vi "water level controller.vi"() -> ()   [LabVIEW 2016]
uses:
  <vilib>/LabVIEW Hacker/LINX/Private/Type Defs/Interface.ctl
  <vilib>/MakerHub/LINX/LMH-LINX.lvlib
  <vilib>/MakerHub/LINX/Public/Sensors/Distance/Ultrasonic/Ultrasonic.lvlib
  <vilib>/LabVIEW Hacker/LINX/Private/Type Defs/User Platform.ctl
  <vilib>/MakerHub/LINX/Public/Utilities/Open Serial.vi
panel:
  in  "Lower Tank level":dbl
  in  "Upper Tank Level":dbl
  out "Centimeters":dbl format="%_1f"
  in  "stop":bool
  out "Tank":dbl(slide) scale=0.0..35.0
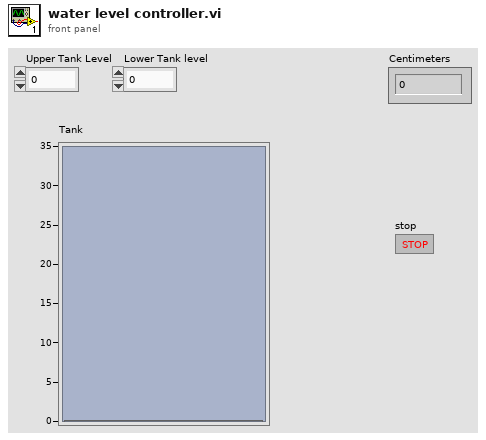
[diagram p1: front panel]
types:
  T1 = typedef "LVH-LINX.lvlib/Interface.ctl" = enum16{"Serial", "TCP"}
  T2 = typedef "LVH-LINX.lvlib/User Platform.ctl" = enum16{"Default", "LINX", "myRIO"}
  T3 = typedef "LMH-LINX.lvlib/LINX Ref.ctl" = cluster{"IO":T4, "Interface":T5, "LINX Device Config":T6}
  T4 = typedef "LMH-LINX.lvlib/Platform.ctl" = enum16{"Remote", "Local"}
  T5 = typedef "LMH-LINX.lvlib/Interface.ctl" = enum16{"Serial", "TCP"}
  T6 = typedef "LMH-LINX.lvlib/Device.lvlib/LINX Device Config.ctl" = cluster{"Interface":T5, "COM Port":refnum<visa-resource-name>, "TCP Configuration":T7, "Device Family":u8, "Device ID":u8, "Device Name":string, "TCP Ref":refnum<k5>, "Channels":T8}
  T7 = typedef "LMH-LINX.lvlib/Device.lvlib/TCP Config.ctl" = cluster{"IP Address":string, "Port":u16}
  T8 = typedef "LMH-LINX.lvlib/Channels.ctl" = cluster{"DI":u8[], "DO":u8[], "AI":u8[], "AO":u8[], "PWM":u8[], "QE":u8[], "UART":u8[], "I2C 2":u8[], "SPI":u8[], "CAN":u8[], "Servo":u8[], "AI Ref (V)":dbl, "AI Resolution (Bits)":u8, "AO Ref (V)":dbl, "AO Resolution (Bits)":u8}
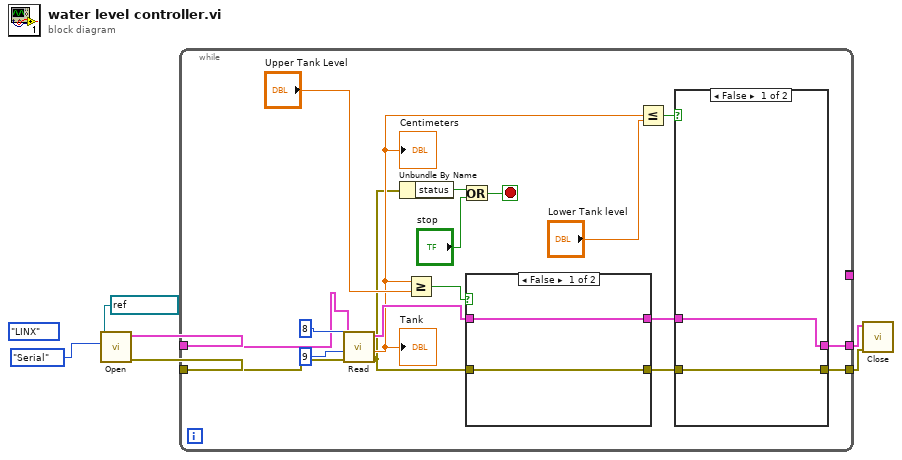
[diagram p0: block diagram]
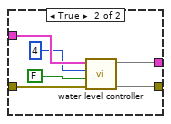
[diagram p2: hidden frame]
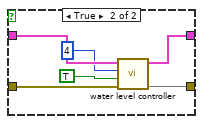
[diagram p3: hidden frame]
diagram:
  (unwired) User_Platform."LINX" ("Platform")
  n1 = call-poly <vilib>:"Open.vi"("Baud Rate Override"=Interface."Serial" ("Interface"), "Serial Port"=refnum<visa-resource-name> "COM23") -> ("Error Out"=w5:errorcluster, "LINX Resource"=w6:T3)  [unwired: 7 in, 1 out]
  n2 = while {
    tunnel: w6 -> [w9]
    tunnel: w5 -> [w8]
    tunnel: [w14] -> w3
    tunnel: [w13] -> w2
    tunnel: [w7] -> _
    tunnel: _ -> [w7]
    stop <- w23 stop-if-true
    n3 = call <vilib>:"Read.vi"("Error In"=w8, "DO Channel"=u8 9 ("Echo Pin (DI)"), "DI Channel"=u8 8 ("Trig"), "LINX Resource"=w9) -> ("Error Out"=w11:errorcluster, "Centimeters"=w12:dbl, "LINX Resource"=w20:T3)  [unwired: 4 in, 1 out]
    "Tank" <- w12
    "Centimeters" <- w12
    n4 = Unbundle By Name(w11) -> ("status"=w25:bool)
    n5 = Greater Or Equal?(x=w12, y="Upper Tank Level") -> (x >= y?=w19:bool)
    n6 = Or(x=w25, y="stop") -> (x .or. y?=w23:bool)
    n7 = case shown="False" w19 {
      tunnel: w20 -> [w35 w41]
      tunnel: w11 -> [w34 w40]
      tunnel: [w35 w37] -> w10
      tunnel: [w34 w36] -> w15
      frame False {
      }
      frame True {
        n8 = call "water level controller.vi"(3:w37, 8:w40, 9:TRUE ("Output Value"), 10:u8 4 ("DO Channel"), 11:w41) -> (0:w36)  [unwired: 6 in]
      }
    }
    n9 = Less Or Equal?(x=w12, y="Lower Tank level") -> (x <= y?=w17:bool)
    n10 = case shown="False" w17 {
      tunnel: w10 -> [w27 w33]
      tunnel: w15 -> [w26 w32]
      tunnel: [w27 w29] -> w14
      tunnel: [w26 w28] -> w13
      frame False {
      }
      frame True {
        n11 = call "water level controller.vi"(8:w32, 9:FALSE ("Output Value"), 10:u8 4 ("DO Channel"), 11:w33) -> (0:w28, 3:w29)  [unwired: 6 in]
      }
    }
  }
  n12 = call <vilib>:"Close.vi"("Error In"=w2, "LINX Resource"=w3) -> ()  [unwired: 9 in, 1 out]
